vi "Reset.vi"(11 "error in (no error)":errorcluster) -> (15 "error out":errorcluster)   [LabVIEW 2024, in "GRBL 1.1.lvlib"]
doc: "Software reset that retain machine position."
uses:
  GRBL 1.1.lvlib
panel:
  out "Limit switch":cluster{"X":bool, "Y":bool, "Z":bool}
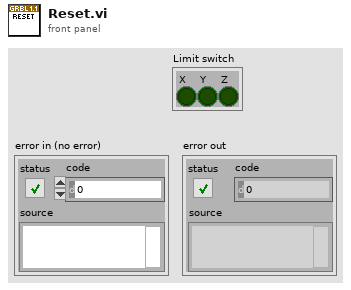
[diagram p1: front panel]
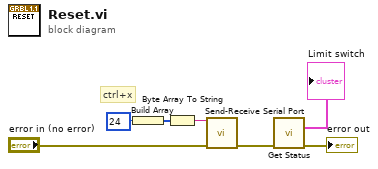
[diagram p0: block diagram]
diagram:
  # "ctrl+x"
  n1 = Build Array(u8 24) -> (w6:u8[])
  n2 = Byte Array To String(unsigned byte array=w6) -> (string=w5:string)
  n3 = call "Send-Receive Serial Port.vi"("Data to write"=w5, "error in (no error)"="error in (no error)") -> ("error out"=w3:errorcluster)  [unwired: 12 in, 1 out]
  n4 = call "Get Status.vi"("error in (no error)"=w3) -> ("Limit switch"=→"Limit switch":cluster{"X":bool, "Y":bool, "Z":bool}, "error out"=→"error out":errorcluster)  [unwired: 10 in, 3 out]
